vi "4.5.vi"() -> ()   [LabVIEW 2017]
panel:
  in  "指定值":dbl
  out "随机数":dbl
  out "循环次数":i32
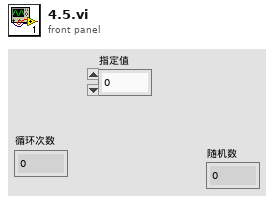
[diagram p1: front panel]
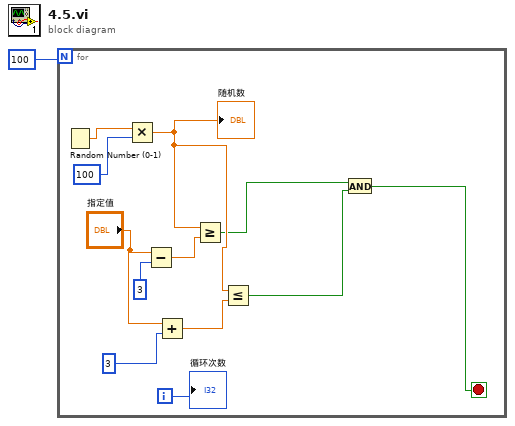
[diagram p0: block diagram]
diagram:
  n1 = for {
    N: 100 -> [_]
    i -> [w13]
    stop <- w10 stop-if-true
    n2 = Random Number (0-1)() -> (number: 0 to 1=w12:dbl)
    n3 = Multiply(x=w12, y=100) -> (x*y=w5:dbl)
    "随机数" <- w5
    n4 = Subtract(x="指定值", y=3) -> (x-y=w8:dbl)
    n5 = Add(x="指定值", y=3) -> (x+y=w4:dbl)
    n6 = Greater Or Equal?(x=w5, y=w8) -> (x >= y?=w2:bool)
    n7 = Less Or Equal?(x=w5, y=w4) -> (x <= y?=w3:bool)
    n8 = And(x=w2, y=w3) -> (x .and. y?=w10:bool)
    "循环次数" <- w13
  }
